vi "lock-in_configure_analysis.vi"(1 "FPGA VI Reference in":T1) -> (0 "FPGA VI Reference Out":T1)   [LabVIEW 2013]
uses:
  fpga-bitfile-ref.ctl
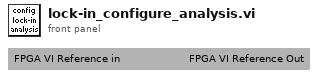
[diagram p1: front panel]
types:
  T1 = typedef "fpga-bitfile-ref.ctl" = refnum<k20>
  T2 = enum8{"NULL", "Data sent to host", "dt/tau", "Voltage range"}
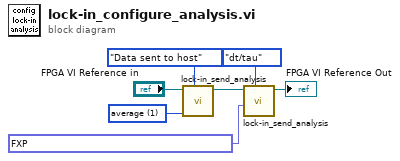
[diagram p0: block diagram]
diagram:
  w6 = u8 1 items=["LI", "average"] ("data sent back")
  n1 = call "lock-in_send_analysis.vi"("order"=T2."Data sent to host", "data sent back"=w6, "FPGA VI Reference In"="FPGA VI Reference in") -> ("FPGA VI Reference Out"=w2:T1)  [unwired: 2 in, 6 out]
  n2 = call "lock-in_send_analysis.vi"("order"=T2."dt/tau", "dt/tau"=fxp<+,32,0> 8.00006091594696e-06, "FPGA VI Reference In"=w2) -> ("FPGA VI Reference Out"=→"FPGA VI Reference Out":T1)  [unwired: 2 in, 6 out]
